vi "Parse Response for Result or Error.vi"(8 "error in":errorcluster, 10 "Response String In":string) -> (0 "error out":errorcluster, 1 "LabVIEW Error?":bool=TRUE, 2 "JSON out":refnum<class "JSON Datatype.lvclass">)   [LabVIEW 2015, in "JSONRPC Server.lvclass"]
uses:
  JSONRPC Server.lvclass
  <vilib>/National Instruments/JSON Support for LabVIEW/JSON Data Classes/JSON Datatype/JSON Datatype.lvclass
  <vilib>/National Instruments/JSON Support for LabVIEW/JSON Parsing/Tokenize  JSON String.vi
  <vilib>/Utility/error.llb/Trim Whitespace.vi
  <vilib>/National Instruments/JSON Support for LabVIEW/JSON Data Classes/JSON Datatype/New JSON.vi
  <vilib>/National Instruments/JSON Support for LabVIEW/JSON Data Classes/JSON Numeric/New JSON Numeric.vi
  <vilib>/National Instruments/JSON Support for LabVIEW/JSON Data Classes/JSON Boolean/New JSON Boolean.vi
  <vilib>/National Instruments/JSON Support for LabVIEW/JSON Data Classes/JSON Null/New JSON Null.vi
  <vilib>/National Instruments/JSON Support for LabVIEW/JSON Parsing/Tokens to String.vi
  <vilib>/National Instruments/JSON Support for LabVIEW/JSON Data Classes/JSON String/New JSON String.vi
  <vilib>/National Instruments/JSON Support for LabVIEW/JSON Parsing/Tokens to Array.vi
  <vilib>/National Instruments/JSON Support for LabVIEW/JSON Parsing/Tokens to Object.vi
  <vilib>/National Instruments/JSON Support for LabVIEW/JSON Data Classes/JSON Datatype/To More Specific Type (Object).vi
  <vilib>/National Instruments/JSON Support for LabVIEW/JSON Data Classes/JSON Object/Get Value (JSON).vi
  <vilib>/National Instruments/JSON Support for LabVIEW/JSON Data Classes/JSON Datatype/To More Specific Type (Numeric).vi
  <vilib>/National Instruments/JSON Support for LabVIEW/JSON Data Classes/JSON Numeric/Read value (Numeric).vi
  <vilib>/National Instruments/JSON Support for LabVIEW/JSON Data Classes/JSON Datatype/To More Specific Type (String).vi
  <vilib>/National Instruments/JSON Support for LabVIEW/JSON Data Classes/JSON String/Read value (String).vi
  <vilib>/National Instruments/JSON Support for LabVIEW/JSON Data Classes/JSON Basic Type/JSON Basic Type.lvclass
  <vilib>/National Instruments/JSON Support for LabVIEW/JSON Data Classes/JSON Numeric/JSON Numeric.lvclass
  <vilib>/National Instruments/JSON Support for LabVIEW/JSON Data Classes/JSON String/JSON String.lvclass
  <vilib>/National Instruments/JSON Support for LabVIEW/JSON Data Classes/JSON Object/JSON Object.lvclass
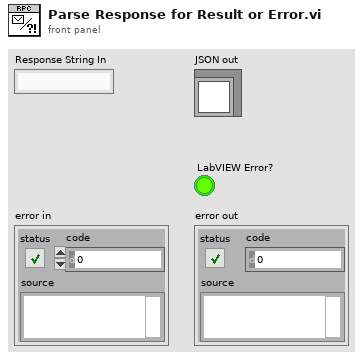
[diagram p1: front panel]
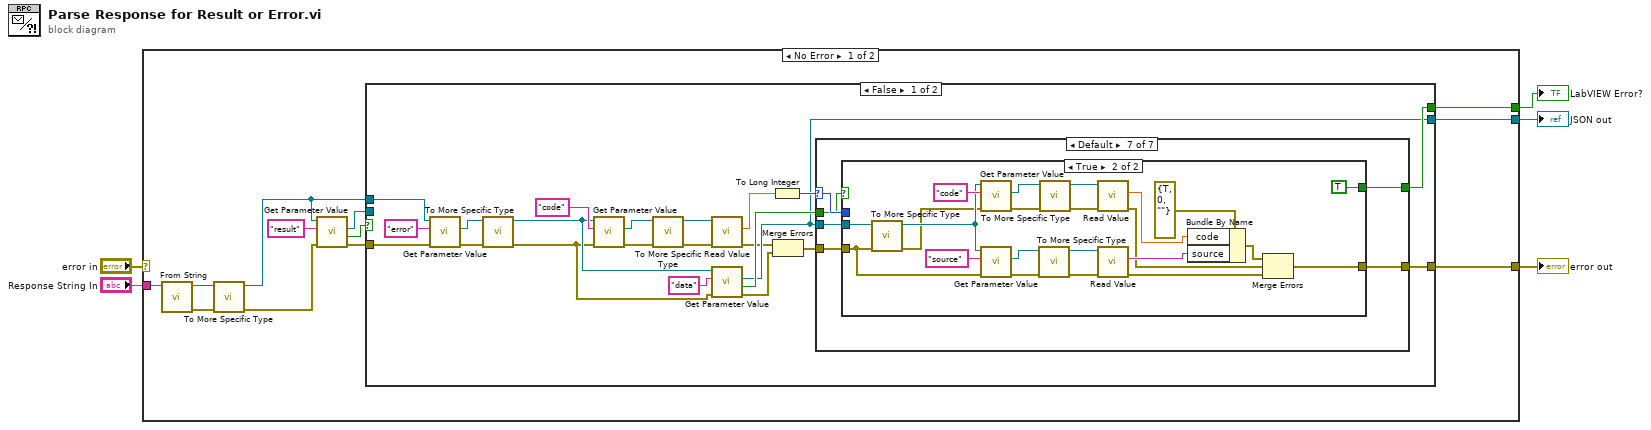
[diagram p0: block diagram]
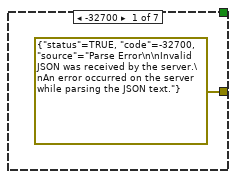
[diagram p2: hidden frame]
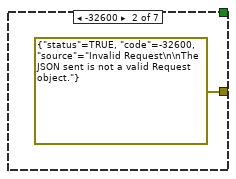
[diagram p3: hidden frame]
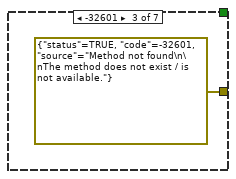
[diagram p4: hidden frame]
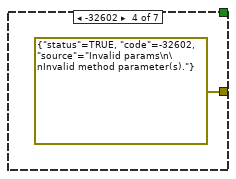
[diagram p5: hidden frame]
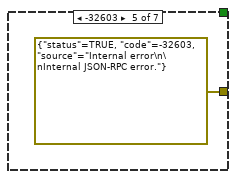
[diagram p6: hidden frame]
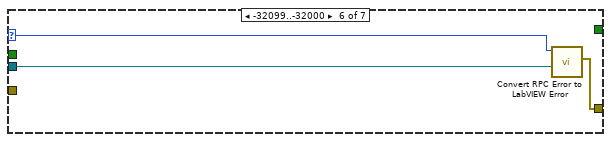
[diagram p7: hidden frame]
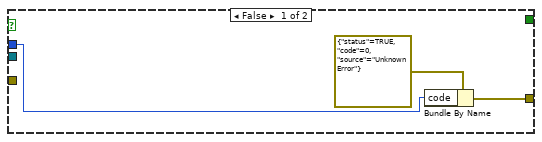
[diagram p8: hidden frame]
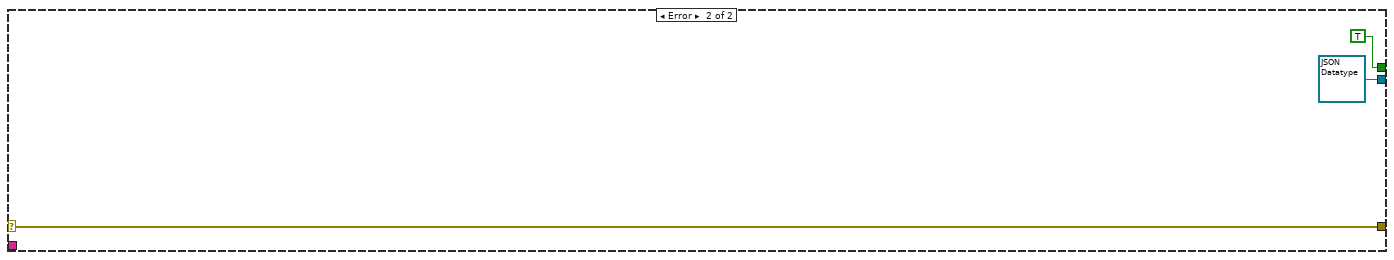
[diagram p10: hidden frame]
diagram:
  n1 = case shown="No Error" "error in" {
    selector: "error in" -> [_ w82]
    tunnel: "Response String In" -> [w14 _]
    tunnel: [w17 refnum<class "JSON Datatype.lvclass"> refnum ("value")] -> w1
    tunnel: [w16 w82] -> w3
    tunnel: [w15 TRUE] -> w2
    frame No Error {
      n2 = call <vilib>:"From String.vi"("JSON String"=w14) -> ("error out"=w13:errorcluster, "JSON out"=w12:refnum<class "JSON Datatype.lvclass">)  [unwired: 9 in]
      n3 = call-poly <vilib>:"To More Specific Type.vi"("error in (no error)"=w13, "JSON Datatype in"=w12) -> ("error out"=w10:errorcluster, "JSON Datatype out"=w8:refnum<class "JSON Object.lvclass">)  [unwired: 8 in]
      n4 = call-poly <vilib>:"Get Parameter Value.vi"("error in (no error)"=w10, "key"="result", "JSON Object in"=w8) -> ("error out"=w6:errorcluster, "found"=w9:bool, "value"=w7:refnum<class "JSON Datatype.lvclass">)  [unwired: 6 in]
      n5 = case shown="False" w9 {
        tunnel: [w30 w80] -> w17
        tunnel: [w38 w79] -> w16
        tunnel: [w37 _] -> w15
        tunnel: w8 -> [w36 _]
        tunnel: w7 -> [_ w80]
        tunnel: w6 -> [w25 w79]
        frame False {
          n6 = call-poly <vilib>:"Get Parameter Value.vi"("error in (no error)"=w25, "key"="error", "JSON Object in"=w36) -> ("error out"=w24:errorcluster, "value"=w34:refnum<class "JSON Datatype.lvclass">)  [unwired: 6 in, 1 out]
          n7 = call-poly <vilib>:"To More Specific Type.vi"("error in (no error)"=w24, "JSON Datatype in"=w34) -> ("error out"=w21:errorcluster, "JSON Datatype out"=w27:refnum<class "JSON Object.lvclass">)  [unwired: 8 in]
          n8 = call-poly <vilib>:"Get Parameter Value.vi"("error in (no error)"=w21, "key"="code", "JSON Object in"=w27) -> ("error out"=w23:errorcluster, "value"=w28:refnum<class "JSON Datatype.lvclass">)  [unwired: 6 in, 1 out]
          n9 = call-poly <vilib>:"To More Specific Type.vi"("error in (no error)"=w23, "JSON Datatype in"=w28) -> ("error out"=w22:errorcluster, "JSON Datatype out"=w29:refnum<class "JSON Numeric.lvclass">)  [unwired: 8 in]
          n10 = call-poly <vilib>:"Read Value.vi"("error in (no error)"=w22, "JSON String in"=w29) -> ("error out"=w20:errorcluster, "value"=w26:dbl)  [unwired: 7 in, 1 out]
          n11 = call-poly <vilib>:"Get Parameter Value.vi"("error in (no error)"=w21, "key"="data", "JSON Object in"=w27) -> ("error out"=w19:errorcluster, "found"=w31:bool, "value"=w30:refnum<class "JSON Datatype.lvclass">)  [unwired: 6 in]
          n12 = To Long Integer(number=w26) -> (32bit integer=w39:i32)
          n13 = Merge Errors(w20, w19) -> (w18:errorcluster)
          n14 = case shown="Default" w39 {
            selector: w39 -> [_ _ _ _ _ w47 w51]
            tunnel: [errorcluster {"status"=TRUE, "code"=-32700, "source"="Parse Error\n\nInvalid JSON was received by the server.\nAn error occurred on the server while parsing the JSON text."} ("error constant") errorcluster {"status"=TRUE, "code"=-32600, "source"="Invalid Request\n\nThe JSON sent is not a valid Request object."} ("error constant") errorcluster {"status"=TRUE, "code"=-32601, "source"="Method not found\n\nThe method does not exist / is not available."} ("error constant") errorcluster {"status"=TRUE, "code"=-32602, "source"="Invalid params\n\nInvalid method parameter(s)."} ("error constant") errorcluster {"status"=TRUE, "code"=-32603, "source"="Internal error\n\nInternal JSON-RPC error."} ("error constant") w45 w53] -> w38
            tunnel: w30 -> [_ _ _ _ _ w46 w52]
            tunnel: [_ _ _ _ _ _ w50] -> w37
            tunnel: w31 -> [_ _ _ _ _ _ w49]
            tunnel: w18 -> [_ _ _ _ _ _ w48]
            frame -32700 {
            }
            frame -32600 {
            }
            frame -32601 {
            }
            frame -32602 {
            }
            frame -32603 {
            }
            frame -32099..-32000 {
              n15 = call "Convert RPC Error to LabVIEW Error.vi"("JSON in"=w46, "RPC Error Code"=w47) -> ("error out"=w45:errorcluster)  [unwired: 9 in]
            }
            frame Default {
              n16 = case shown="True" w49 {
                tunnel: [w54 w57] -> w53
                tunnel: w52 -> [_ w76]
                tunnel: w51 -> [w55 _]
                tunnel: [_ TRUE] -> w50
                tunnel: w48 -> [_ w61]
                frame False {
                  n17 = Bundle By Name(cluster=errorcluster {"status"=TRUE, "code"=0, "source"="Unknown Error"} ("error constant"), "code"=w55) -> (w54:errorcluster)
                }
                frame True {
                  n18 = call-poly <vilib>:"To More Specific Type.vi"("error in (no error)"=w61, "JSON Datatype in"=w76) -> ("error out"=w66:errorcluster, "JSON Datatype out"=w69:refnum<class "JSON Object.lvclass">)  [unwired: 8 in]
                  n19 = call-poly <vilib>:"Get Parameter Value.vi"("error in (no error)"=w66, "key"="code", "JSON Object in"=w69) -> ("error out"=w65:errorcluster, "value"=w75:refnum<class "JSON Datatype.lvclass">)  [unwired: 6 in, 1 out]
                  n20 = call-poly <vilib>:"Get Parameter Value.vi"("error in (no error)"=w61, "key"="source" ("Parameter Name"), "JSON Object in"=w69) -> ("error out"=w63:errorcluster, "value"=w70:refnum<class "JSON Datatype.lvclass">)  [unwired: 6 in, 1 out]
                  n21 = call-poly <vilib>:"To More Specific Type.vi"("error in (no error)"=w63, "JSON Datatype in"=w70) -> ("error out"=w62:errorcluster, "JSON Datatype out"=w71:refnum<class "JSON String.lvclass">)  [unwired: 8 in]
                  n22 = call-poly <vilib>:"To More Specific Type.vi"("error in (no error)"=w65, "JSON Datatype in"=w75) -> ("error out"=w64:errorcluster, "JSON Datatype out"=w74:refnum<class "JSON Numeric.lvclass">)  [unwired: 8 in]
                  n23 = call-poly <vilib>:"Read Value.vi"("error in (no error)"=w64, "JSON String in"=w74) -> ("error out"=w60:errorcluster, "value"=w72:dbl)  [unwired: 7 in, 1 out]
                  n24 = call-poly <vilib>:"Read Value.vi"("error in (no error)"=w62, "JSON String in"=w71) -> ("error out"=w59:errorcluster, "value"=w67:string)  [unwired: 7 in, 1 out]
                  n25 = Bundle By Name(cluster=errorcluster {"status"=TRUE, "code"=0, "source"=""} ("error constant"), "code"=w72, "source"=w67) -> (w58:errorcluster)
                  n26 = Merge Errors(w58, w60, w59) -> (w57:errorcluster)
                }
              }
            }
          }
        }
        frame True {
        }
      }
    }
    frame Error {
    }
  }
  "error out" <- w3
  "JSON out" <- w1
  "LabVIEW Error?" <- w2
